vi "InitiateGeneration.vi"(8 "error in (no error)":errorcluster, 11 "ClassIn":refnum<class "Keysight335XX.lvclass">) -> (0 "error out":errorcluster, 3 "ClassOut":refnum<class "Keysight335XX.lvclass">)   [LabVIEW 2014, in "FGenPlugins.lvlib" / "Keysight335XX.lvclass"]
uses:
  Keysight335XX.lvclass
  MyPluginBaseClass/TypeDef/ChannelParamElement.ctl
  MyPluginBaseClass/NISTFGenPluginsBase.lvclass
  <instrlib>/Agilent 3352X Series/Agilent 3352X Series.lvlib
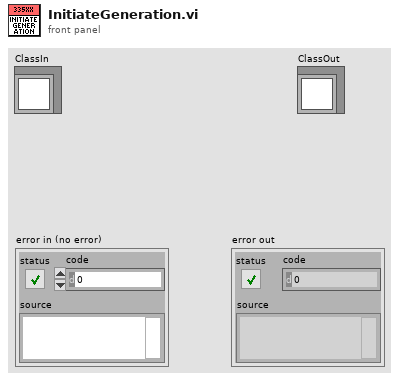
[diagram p1: front panel]
types:
  T1 = typedef "FGenPlugins.lvlib/NISTFGenPluginsBase.lvclass/ChannelParamElement.ctl" = cluster{"sName":string, "eOperateMode":u16, "bEnabled":bool, "eOutputMode":u16, "iIndex":i32, "iNameBufferSize":i32, "fGain":dbl}
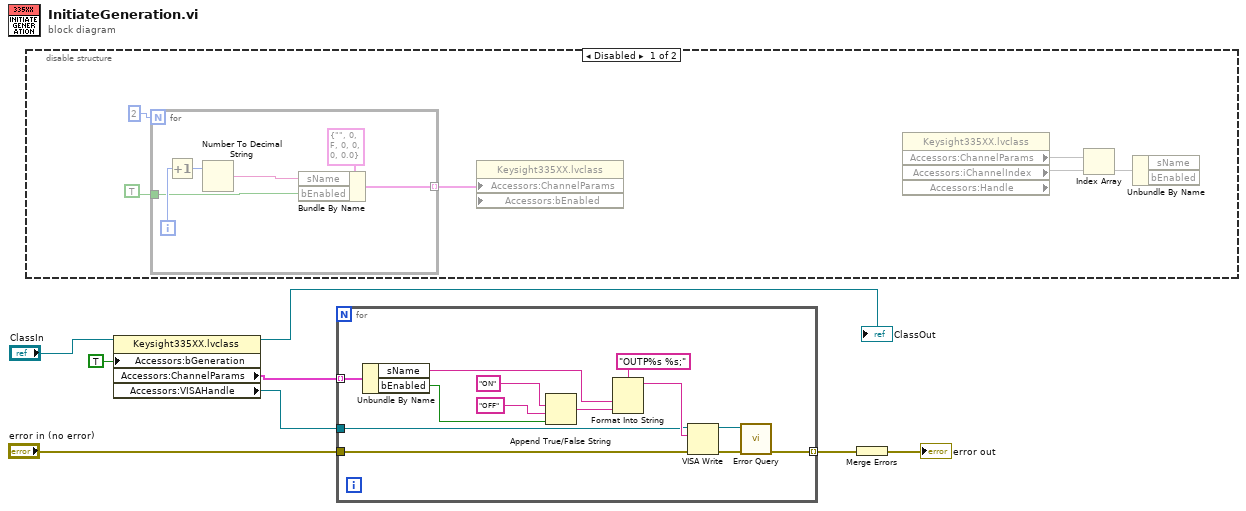
[diagram p0: block diagram]
diagram:
  n1 = disable-structure shown="Disabled" {
    frame Disabled {
      n2 = for {
        N: 2 -> [_]
        tunnel: TRUE -> [w16]
        tunnel: [w17] -> w9 mode=indexing
        i -> [w20]
        n3 = Increment(x=w20) -> (x+1=w19:i32)
        n4 = Number To Decimal String(number=w19) -> (decimal integer string=w15:string)  [unwired: 1 in]
        n5 = Bundle By Name(cluster=T1 {"sName"="", "eOperateMode"=0, "bEnabled"=FALSE, "eOutputMode"=0, "iIndex"=0, "iNameBufferSize"=0, "fGain"=0.0} ("ChannelParamElement"), "sName"=w15, "bEnabled"=w16) -> (w17:T1)
      }
      n6 = property class="Keysight335XX.lvclass" props=["Accessors:ChannelParams", "Accessors:bEnabled"]("Accessors:ChannelParams"=w9) -> ()  [unwired: 3 in, 2 out]
      n7 = property class="Keysight335XX.lvclass" props=["Accessors:ChannelParams", "Accessors:iChannelIndex", "Accessors:Handle"]() -> ("Accessors:ChannelParams"=w12, "Accessors:iChannelIndex"=w10)  [unwired: 2 in, 3 out]
      n8 = Index Array(array=w12, index=w10) -> (element=w11)
      n9 = Unbundle By Name(w11) -> ()  [unwired: 2 out]
    }
    frame Enabled {
    }
  }
  n10 = property class="Keysight335XX.lvclass"(reference="ClassIn", "Accessors:bGeneration"=TRUE ("bGeneration")) -> (reference out=→"ClassOut":refnum<class "Keysight335XX.lvclass">, "Accessors:ChannelParams"=w5:T1[], "Accessors:VISAHandle"=w4:refnum<visa-resource-name>)  [unwired: 1 in, 1 out]
  n11 = for {
    tunnel: w5 -> [w33] mode=indexing
    tunnel: w4 -> [w24]
    tunnel: "error in (no error)" -> [w23]
    tunnel: [w21] -> w2 mode=indexing
    n12 = Unbundle By Name(w33) -> ("sName"=w26:string, "bEnabled"=w25:bool)
    n13 = Append True/False String(1:w25, 2:"OFF", 3:"ON") -> (0:w27:string)  [unwired: 1 out]
    n14 = Format Into String(format string="OUTP%s %s;", w26, w27) -> (resulting string=w29:string)  [unwired: 2 in, 1 out]
    n15 = VISA Write(VISA resource name=w24, write buffer=w29, error in (no error)=w23) -> (VISA resource name out=w30:refnum<visa-resource-name>, error out=w22:errorcluster)  [unwired: 1 out]
    n16 = call <instrlib>:"Error Query.vi"("error in (no error)"=w22, "VISA resource name"=w30) -> ("error out"=w21:errorcluster)  [unwired: 9 out]
  }
  n17 = Merge Errors(w2) -> (→"error out":errorcluster)
